vi "TRAJECTORY_EXECUTE_REVERSE_OLD.vi"(5 "Wheel Base FT":dbl, 6 "RamseteEnable":bool=TRUE, 7 "Max Speed\nFT/SEC":dbl, 8 "Init":bool, 9 "Gyro Continous\n (inc counterclockwise)":dbl, 10 "Right Distance":dbl, 11 "Left Distance":dbl) -> (0 "AtReference":bool, 1 "Right Speed Target":dbl, 2 "Left Speed Target":dbl, 3 "outRAMSETE (SI)":T5={"B"=2.0, "Zeta"=0.7, "poseTolerance"={"TRANSLATION"={"X"=0.0, "Y"=0.0}, "ROTATION"={"VALUE"=0.0, "COS"=1.0, "SIN"=0.0}}, "poseError"={"TRANSLATION"={"X"=0.0, "Y"=0.0}, "ROTATION"={"VALUE"=0.0, "COS"=1.0, "SIN"=0.0}}, "Enabled"=TRUE} {"poseError"."ROTATION"."SIN" format="%13.4f"; "poseError"."ROTATION"."COS" format="%13.4f"; "poseError"."ROTATION"."VALUE" format="%13.4f"; "poseError"."TRANSLATION"."Y" format="%14.3f"; "poseError"."TRANSLATION"."X" format="%14.3f"; "poseTolerance"."ROTATION"."SIN" format="%13.4f"; "poseTolerance"."ROTATION"."COS" format="%13.4f"; "poseTolerance"."ROTATION"."VALUE" format="%13.4f"; "poseTolerance"."TRANSLATION"."Y" format="%14.3f"; "poseTolerance"."TRANSLATION"."X" format="%14.3f"; "Zeta" format="%12.3f"; "B" format="%12.3f"}, 4 "OutputTRAJ_STATE (SI)":T1={"TimeSeconds"=0.0, "Velocity"=0.0, "Acceleration"=0.0, "POSE"={"TRANSLATION"={"X"=0.0, "Y"=0.0}, "ROTATION"={"VALUE"=0.0, "COS"=1.0, "SIN"=0.0}}, "Curvature"=0.0} {"POSE"."ROTATION"."SIN" format="%13.4f"; "POSE"."ROTATION"."COS" format="%13.4f"; "POSE"."ROTATION"."VALUE" format="%13.4f"; "POSE"."TRANSLATION"."Y" format="%14.3f"; "POSE"."TRANSLATION"."X" format="%14.3f"})   [LabVIEW 2019]
uses:
  <vilib>/Rock Robotics/WPI/ThirdParty/JAS_Junk/TrajLib/RAMSETE.ctl
  <vilib>/Rock Robotics/WPI/ThirdParty/JAS_Junk/TrajLib/POSE2D.ctl
  <vilib>/Rock Robotics/WPI/ThirdParty/JAS_Junk/TrajLib/TRANSLATION2D.ctl
  <vilib>/Rock Robotics/WPI/ThirdParty/JAS_Junk/TrajLib/ROTATION2D.ctl
  <vilib>/Rock Robotics/WPI/ThirdParty/JAS_Junk/TrajLib/TRAJ_STATE.ctl
  <vilib>/Rock Robotics/WPI/ThirdParty/JAS_Junk/TrajLib/Rotation_CreateAngle.vi
  <vilib>/Rock Robotics/WPI/ThirdParty/JAS_Junk/TrajLib/Translation_Create.vi
  <vilib>/Rock Robotics/WPI/ThirdParty/JAS_Junk/TrajLib/Trajectory_Library.lvlib
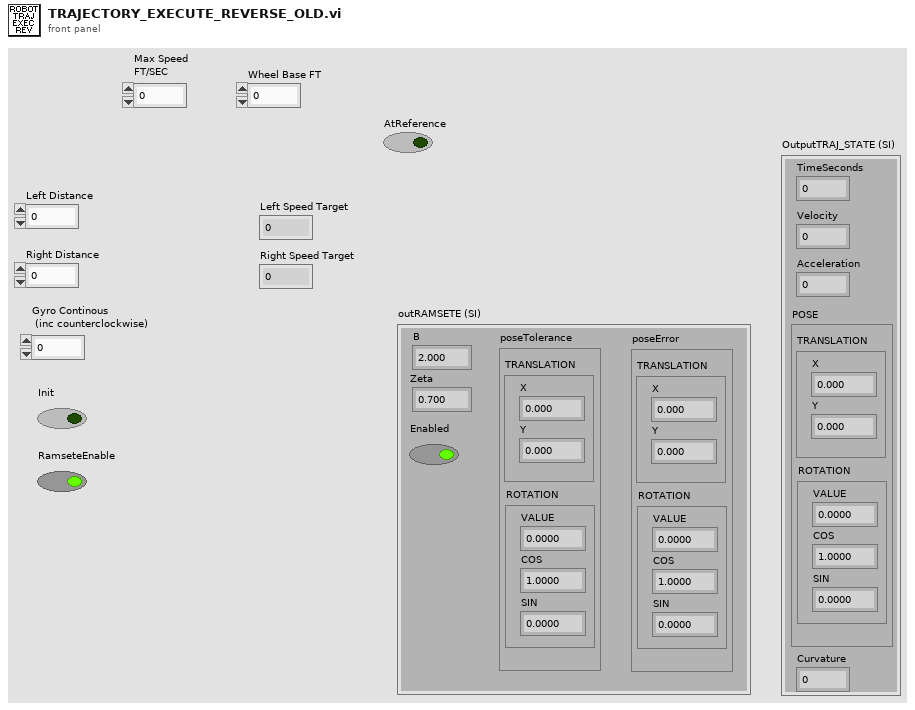
[diagram p1: front panel]
types:
  T1 = typedef "Trajectory_Library.lvlib/TRAJ_STATE.ctl" = cluster{"TimeSeconds":dbl, "Velocity":dbl, "Acceleration":dbl, "POSE":T2, "Curvature":dbl}
  T2 = typedef "Trajectory_Library.lvlib/POSE2D.ctl" = cluster{"TRANSLATION":T3, "ROTATION":T4}
  T3 = typedef "Trajectory_Library.lvlib/TRANSLATION2D.ctl" = cluster{"X":dbl, "Y":dbl}
  T4 = typedef "Trajectory_Library.lvlib/ROTATION2D.ctl" = cluster{"VALUE":dbl, "COS":dbl, "SIN":dbl}
  T5 = typedef "Trajectory_Library.lvlib/RAMSETE.ctl" = cluster{"B":dbl, "Zeta":dbl, "poseTolerance":T2, "poseError":T2, "Enabled":bool}
  T6 = typedef "Trajectory_Library.lvlib/TRAJECTORY.ctl" = cluster{"TotalTImeSecs":dbl, "States":T1[]}
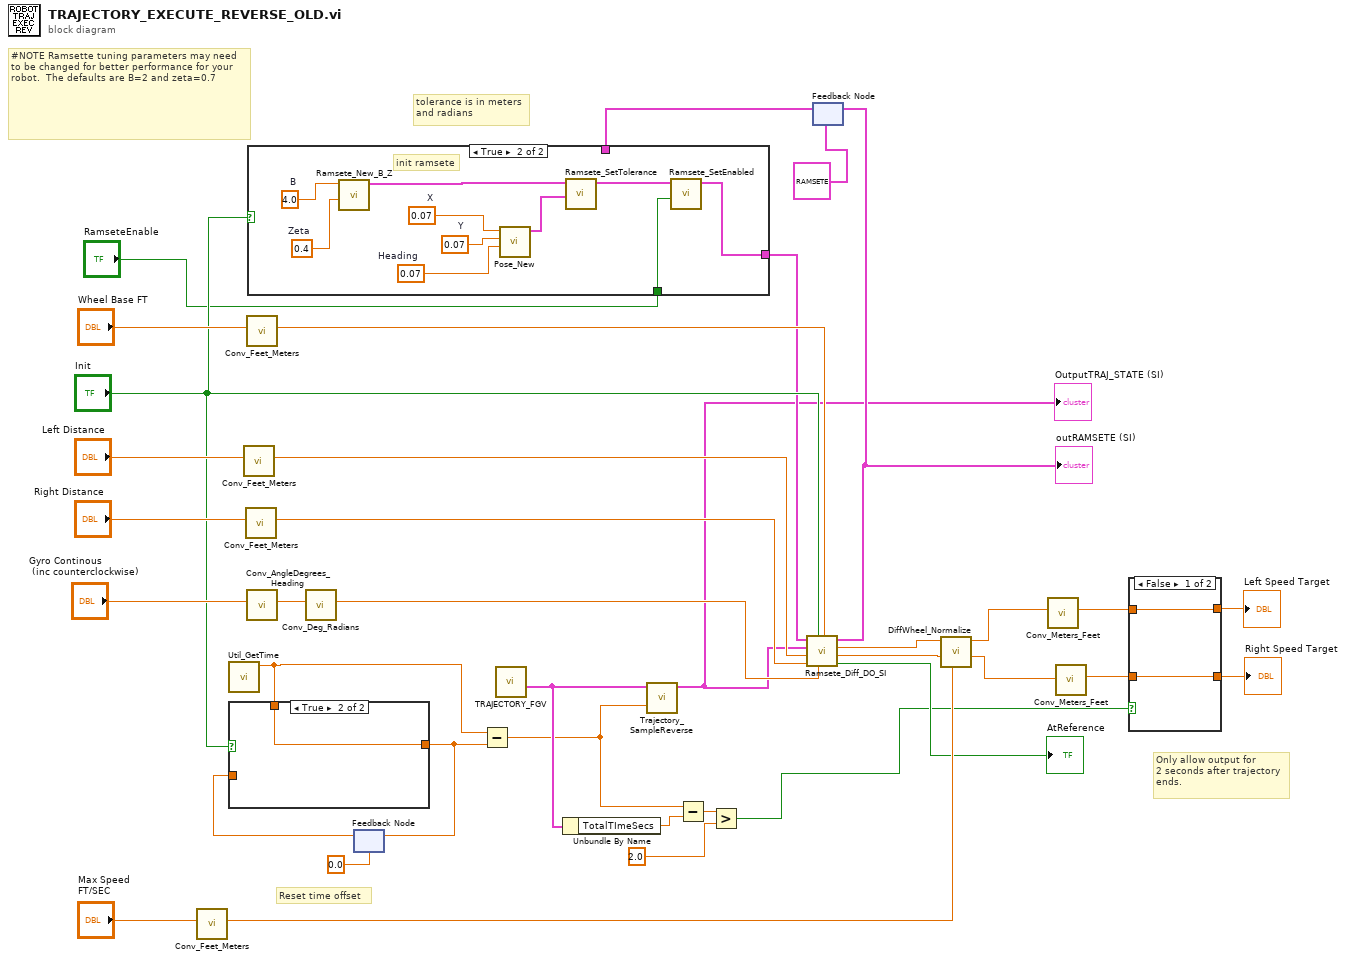
[diagram p0: block diagram]
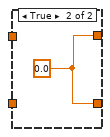
[diagram p3: hidden frame]
diagram:
  # "tolerance is in meters\nand radians"
  # "#NOTE Ramsette tuning parameters may need to be changed for better performance for your robot.  The defaults are B=2 and zeta=0.7"
  # "Only allow output for\n2 seconds after trajectory\nends."
  # "Reset time offset"
  n1 = call <vilib>:"Conv_Feet_Meters.vi"("Feet"="Max Speed\nFT/SEC") -> ("Meters"=w27:dbl)  [unwired: 10 in]
  n2 = call <vilib>:"Util_GetTime.vi"() -> ("FPGA_Time_Seconds"=w2:dbl)  [unwired: 10 in, 1 out]
  n3 = call <vilib>:"Conv_Feet_Meters.vi"("Feet"="Left Distance") -> ("Meters"=w12:dbl)  [unwired: 10 in]
  n4 = call <vilib>:"Conv_Feet_Meters.vi"("Feet"="Right Distance") -> ("Meters"=w11:dbl)  [unwired: 10 in]
  n5 = call <vilib>:"Conv_Feet_Meters.vi"("Feet"="Wheel Base FT") -> ("Meters"=w9:dbl)  [unwired: 10 in]
  n6 = call <vilib>:"Conv_AngleDegrees_Heading.vi"("Degrees"="Gyro Continous\n (inc counterclockwise)") -> ("Heading Degrees"=w23:dbl)  [unwired: 10 in]
  n7 = call <vilib>:"Conv_Deg_Radians.vi"("Degress"=w23) -> ("Radians"=w10:dbl)  [unwired: 10 in]
  n8 = feedback #1(0.0 ("TIME")) -> (w36:dbl)
  n9 = case shown="True" "Init" {
    tunnel: [w38 w39] -> w35
    tunnel: w36 -> [w38 _]
    tunnel: w2 -> [_ w39]
    frame False {
    }
    frame True {
    }
  }
  n10 = feedback-in #1(w35) -> ()
  n11 = Subtract(x=w2, y=w35) -> (x-y=w20:dbl)
  n12 = call "TRAJECTORY_FGV.vi"() -> ("outTRAJECTORY"=w22:T6)  [unwired: 11 in]
  n13 = Unbundle By Name(w22) -> ("TotalTImeSecs"=w21:dbl)
  n14 = call <vilib>:"Trajectory_SampleReverse.vi"("Time"=w20, "InputTRAJECTORY"=w22) -> ("OutputTRAJ_STATE"=w3:T1)  [unwired: 9 in]
  "OutputTRAJ_STATE (SI)" <- w3
  n15 = Subtract(x=w20, y=w21) -> (x-y=w19:dbl)
  n16 = Greater?(x=w19, y=2.0) -> (0:w17:bool)
  n17 = feedback #2(T5 {"B"=2.0, "Zeta"=0.7, "poseTolerance"={"TRANSLATION"={"X"=0.0, "Y"=0.0}, "ROTATION"={"VALUE"=0.0, "COS"=1.0, "SIN"=0.0}}, "poseError"={"TRANSLATION"={"X"=0.0, "Y"=0.0}, "ROTATION"={"VALUE"=0.0, "COS"=1.0, "SIN"=0.0}}, "Enabled"=TRUE} ("RAMSETE")) -> (w6:T5)
  n18 = case shown="True" "Init" {
    tunnel: w6 -> [w40 _]
    tunnel: [w40 w48] -> w5
    tunnel: "RamseteEnable" -> [_ w41]
    frame False {
    }
    frame True {
      w42 = 0.4  # Zeta
      w43 = 4.0  # B
      w44 = 0.07  # Heading
      w45 = 0.07  # Y
      w46 = 0.07  # X
      # "init ramsete"
      n19 = call <vilib>:"Ramsete_New_B_Z.vi"("Zeta"=w42, "B"=w43) -> ("outRAMSETE"=w50:T5)  [unwired: 9 in]
      n20 = call <vilib>:"Pose_New.vi"("Heading"=w44, "Y"=w45, "X"=w46) -> ("out POSe"=w47:T2)  [unwired: 8 in]
      n21 = call <vilib>:"Ramsete_SetTolerance.vi"("tolerancePose"=w47, "inRAMSETE"=w50) -> ("outRAMSETE"=w49:T5)  [unwired: 9 in]
      n22 = call <vilib>:"Ramsete_SetEnabled.vi"("Enabled"=w41, "inRAMSETE"=w49) -> ("outRAMSETE"=w48:T5)  [unwired: 9 in]
    }
  }
  n23 = call <vilib>:"Ramsete_Diff_DO_SI.vi"("WheelBase-Meters"=w9, "Gyro-Radians"=w10, "Reset"="Init", "RightDist-Meters"=w11, "LeftDist-Meters"=w12, "TRAJ_STATE"=w3, "inRAMSETE"=w5) -> ("AtReference"=→"AtReference":bool, "RightVelDmd"=w28:dbl, "LeftVelDmd"=w29:dbl, "outRAMSETE"=w7:T5)  [unwired: 1 out]
  "outRAMSETE (SI)" <- w7
  n24 = feedback-in #2(w7) -> ()
  n25 = call <vilib>:"DiffWheel_Normalize.vi"("Max Speed"=w27, "Right Wheel Demand"=w28, "Left Wheel Demand"=w29) -> ("Normalized Right Wheel Demand"=w24:dbl, "Normalized Left Wheel Demand"=w25:dbl)  [unwired: 7 in]
  n26 = call <vilib>:"Conv_Meters_Feet.vi"("Meters"=w25) -> ("Feet"=w14:dbl)  [unwired: 10 in]
  n27 = call <vilib>:"Conv_Meters_Feet.vi"("Meters"=w24) -> ("Feet"=w13:dbl)  [unwired: 10 in]
  n28 = case shown="False" w17 {
    tunnel: [w52 w53] -> w16
    tunnel: [w51 w53] -> w15
    tunnel: w14 -> [w52 _]
    tunnel: w13 -> [w51 _]
    frame False {
    }
    frame True {
      w53 = 0.0
    }
  }
  "Left Speed Target" <- w16
  "Right Speed Target" <- w15
